vi "PeriodicFilter-Remove invalid Entry.vi"(7 "seconds since 1Jan1904 2":timestamp, 8 "Settings":T1={"threashold(#/s)"=1.0, "Check Peroid(s)"=1.0}, 11 "data in":T3 {"LastCheckT" format="%<%.3X>T"}) -> (0 "removed info":T2[](array[typedef]), 3 "data out":T3 {"LastCheckT" format="%<%.3X>T"})   [LabVIEW 2017, in "Communicable State Machine.lvlib"]
uses:
  Communicable State Machine.lvlib
  Periodic String Filter Data.ctl
  Periodic String Filter Info.ctl
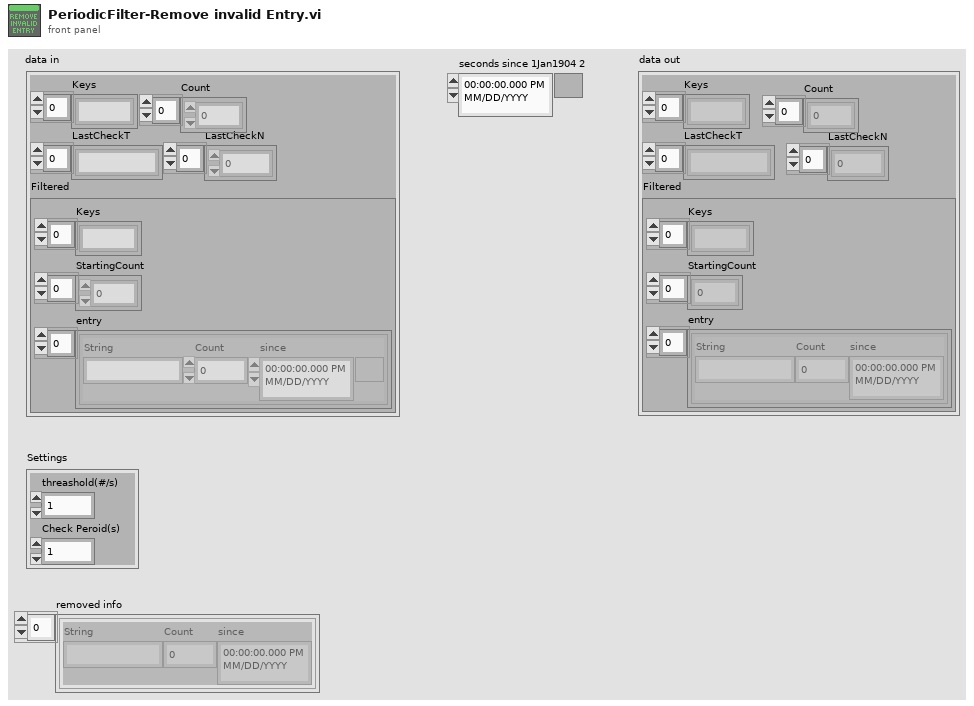
[diagram p1: front panel]
types:
  T1 = cluster{"threashold(#/s)":dbl, "Check Peroid(s)":dbl}
  T2 = typedef "Communicable State Machine.lvlib/Periodic String Filter Info.ctl" = cluster{"String":string, "Count":i64, "since":timestamp}
  T3 = typedef "Communicable State Machine.lvlib/Periodic String Filter Data.ctl" = cluster{"Keys":string[], "Count":i64[], "LastCheckT":timestamp[], "LastCheckN":i64[], "Filtered":cluster{"Keys":string[], "StartingCount":i64[], "entry":T2[]}}
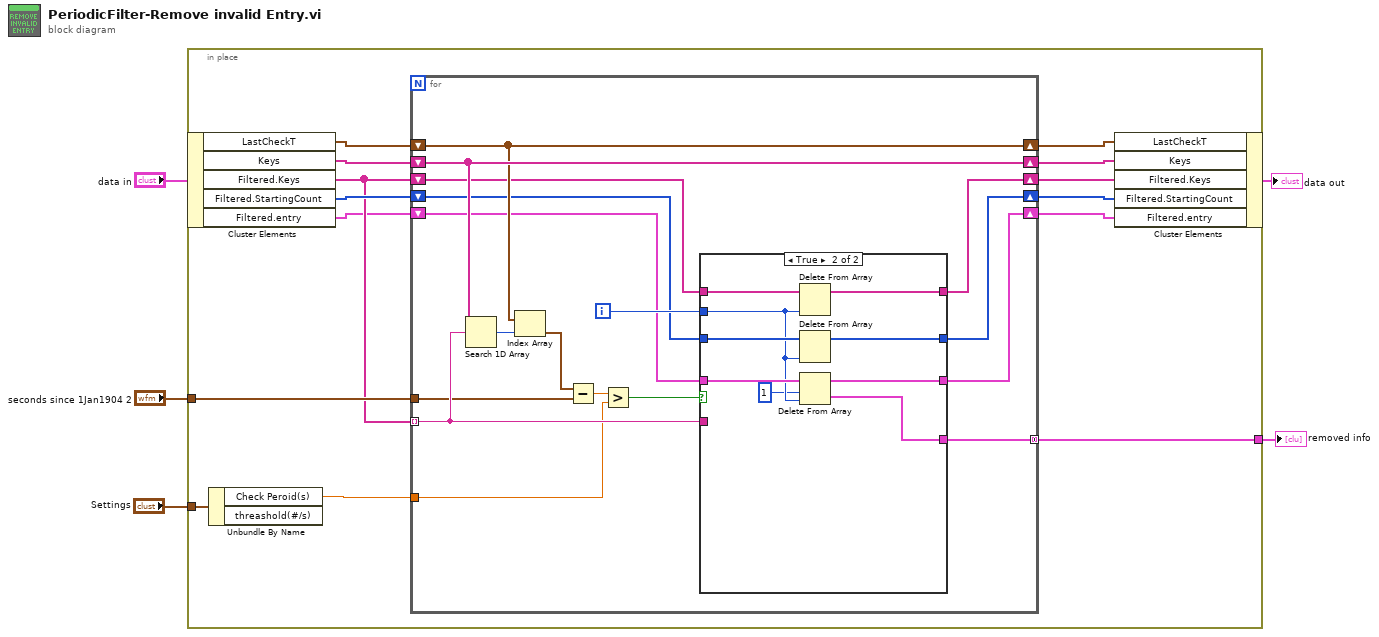
[diagram p0: block diagram]
diagram:
  n1 = in-place "In Place Element Structure" {
    in-place-border: "seconds since 1Jan1904 2" -> [w14]
    in-place-border: [w15] -> w2
    in-place-border: "Settings" -> [w13]
    n2 = in-place-cluster #1("data in") -> ("LastCheckT"=w17:timestamp[], "Keys"=w19:string[], "Filtered.Keys"=w11:string[], "Filtered.StartingCount"=w12:i64[], "Filtered.entry"=w9:T2[])
    n3 = Unbundle By Name(w13) -> ("Check Peroid(s)"=w6:dbl)  [unwired: 1 out]
    n4 = for {
      tunnel: w11 -> [w35] mode=indexing
      shift-right: [w33] -> w18
      shift-left: w19 -> [w33]
      tunnel: [w34] -> w15 mode=concatenating
      shift-right: [w32] -> w16
      shift-left: w17 -> [w32]
      tunnel: w14 -> [w30]
      shift-right: [w21] -> w7
      shift-left: w12 -> [w22]
      shift-right: [w20] -> w10
      shift-left: w11 -> [w27]
      shift-right: [w23] -> w8
      shift-left: w9 -> [w24]
      tunnel: w6 -> [w28]
      i -> [w26]
      n5 = Search 1D Array(1D array=w33, element=w35) -> (index of element=w36:i32)  [unwired: 1 in]
      n6 = Index Array(array=w32, index=w36) -> (element=w31:timestamp)
      n7 = Subtract(x=w31, y=w30) -> (x-y=w29:dbl)
      n8 = Greater?(x=w29, y=w28) -> (0:w25:bool)
      n9 = case shown="True" w25 {
        tunnel: w35 -> [_ _]
        tunnel: [_ w41] -> w34
        tunnel: w27 -> [w37 w48]
        tunnel: w26 -> [_ w45]
        tunnel: w22 -> [w38 w47]
        tunnel: w24 -> [w39 w46]
        tunnel: [w39 w44] -> w23
        tunnel: [w38 w43] -> w21
        tunnel: [w37 w42] -> w20
        frame False {
        }
        frame True {
          n10 = Delete From Array(array=w48, index=w45) -> (array with subset deleted=w42:string[])  [unwired: 1 in, 1 out]
          n11 = Delete From Array(array=w47, index=w45) -> (array with subset deleted=w43:i64[])  [unwired: 1 in, 1 out]
          n12 = Delete From Array(array=w46, length=1, index=w45) -> (deleted portion=w41:T2[], array with subset deleted=w44:T2[])
        }
      }
    }
    n13 = in-place-cluster #1("LastCheckT"=w16, "Keys"=w18, "Filtered.Keys"=w10, "Filtered.StartingCount"=w7, "Filtered.entry"=w8) -> (→"data out":T3)
  }
  "removed info" <- w2
